vi "Set Controls from String Formats_ArrayInputs_SignalingValue.vi"(4 "Defer Panel Updates (T)":bool=TRUE, 6 "Disabled":u8[](array[numeric]), 7 "milliseconds to wait (10 ms)":u32=10, 8 "error in (no error)":errorcluster, 9 "Values":string[](array[string]), 10 "Labels":string[](array[string]), 11 "VI Server Cluster":T1) -> (0 "error out":errorcluster, 3 "VI Server Cluster.DUP":T1)   [LabVIEW 2020, in "VI Server Toolkit LV2013.lvlib"]
doc: "Set multiple Controls Value from string format and converts string values of the selected GUI objects onto original data type."
uses:
  VI Server Toolkit LV2013.lvlib
  VI Server_TypeDefs/VI Server_RefsCluster.ctl
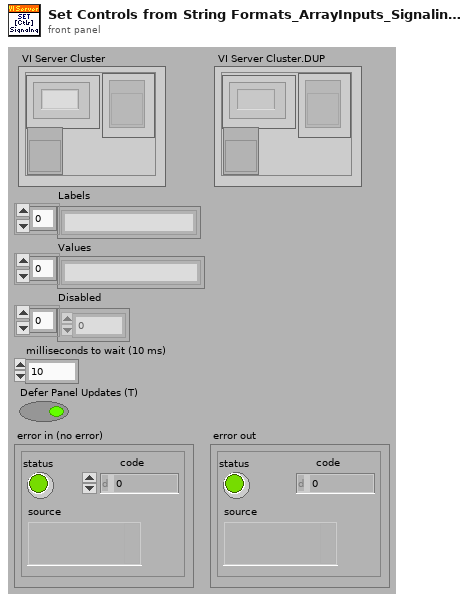
[diagram p1: front panel]
types:
  T1 = typedef "VI Server_RefsCluster.ctl" = cluster{"Labels":string[], "Refs":refnum<vi>[], "VI Ref":refnum<vi>}
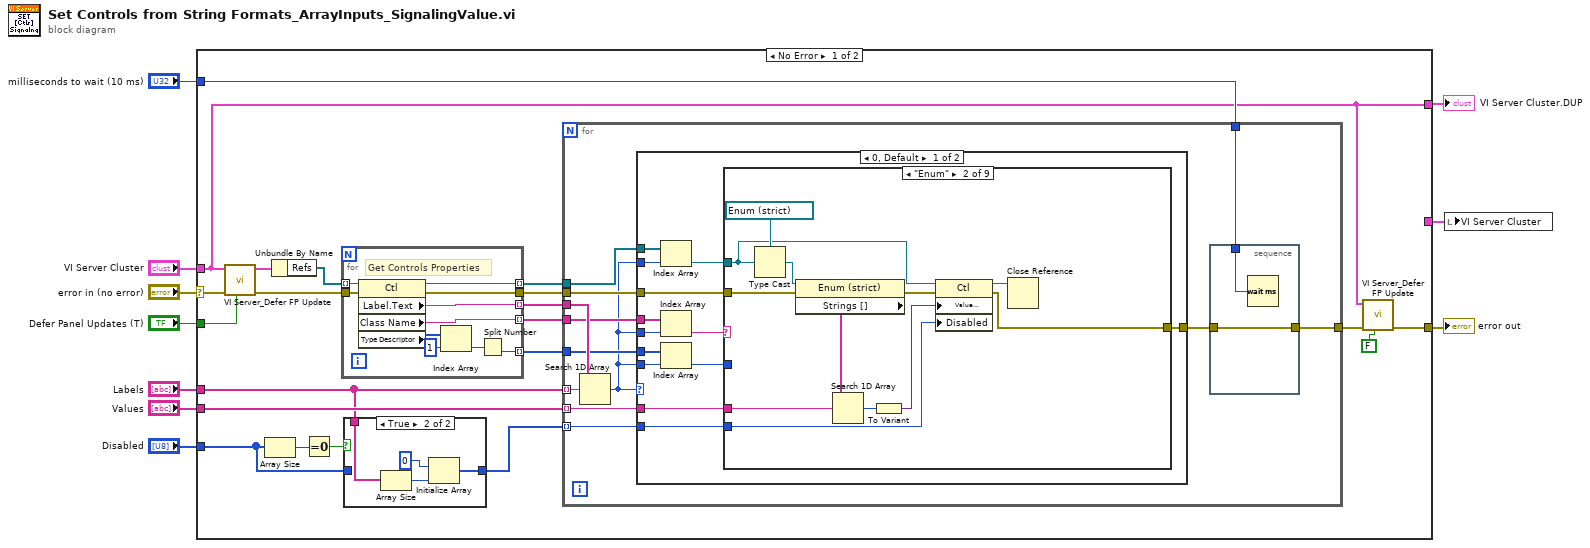
[diagram p0: block diagram]
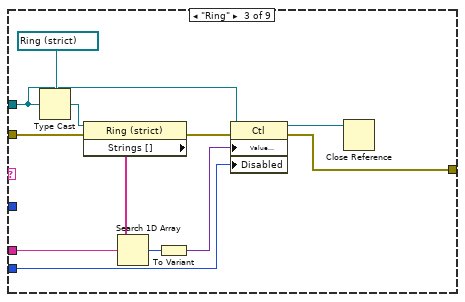
[diagram p4: hidden frame]
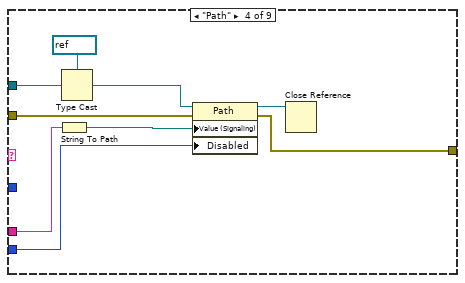
[diagram p5: hidden frame]
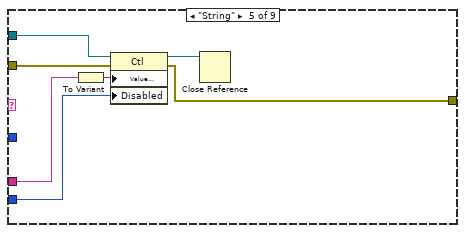
[diagram p6: hidden frame]
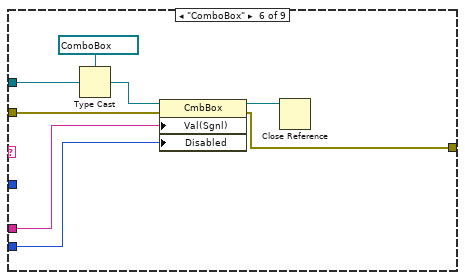
[diagram p7: hidden frame]
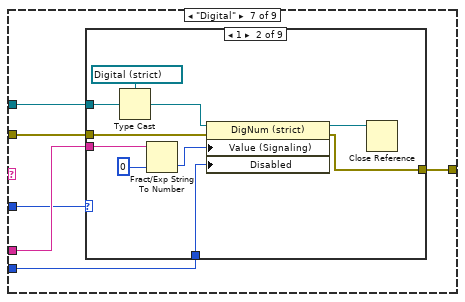
[diagram p8: hidden frame]
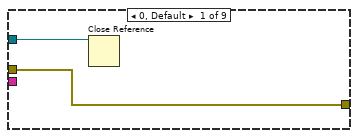
[diagram p9: hidden frame]
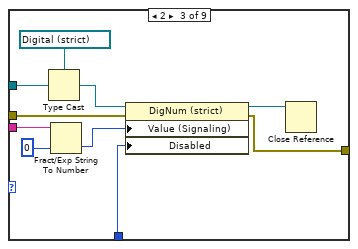
[diagram p10: hidden frame]
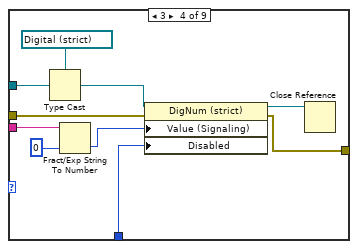
[diagram p11: hidden frame]
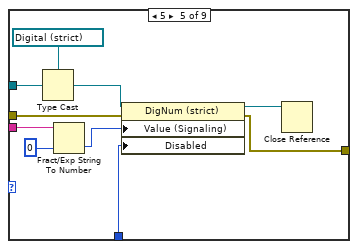
[diagram p12: hidden frame]
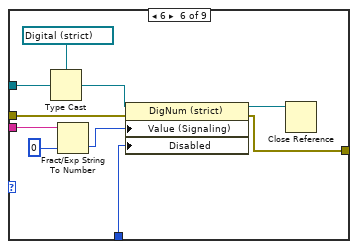
[diagram p13: hidden frame]
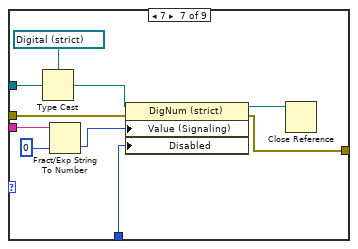
[diagram p14: hidden frame]
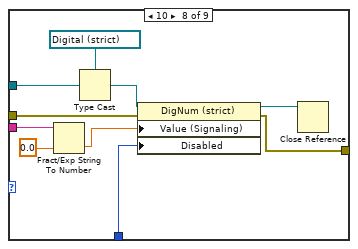
[diagram p15: hidden frame]
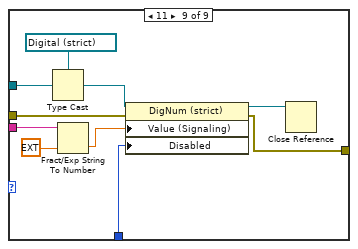
[diagram p16: hidden frame]
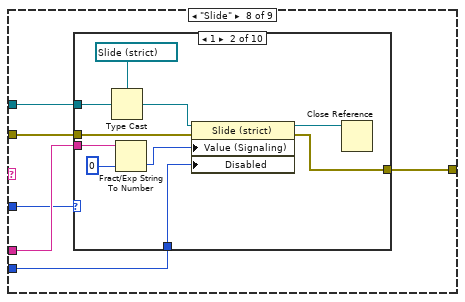
[diagram p17: hidden frame]
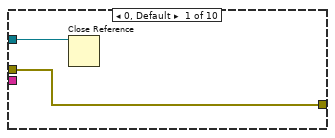
[diagram p18: hidden frame]
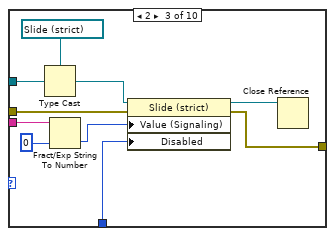
[diagram p19: hidden frame]
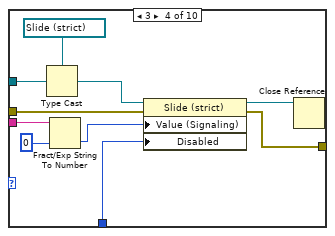
[diagram p20: hidden frame]
diagram:
  n1 = case shown="No Error" "error in (no error)" {
    selector: "error in (no error)" -> [w19 w324]
    tunnel: "Labels" -> [w21 _]
    tunnel: "Disabled" -> [w31 _]
    tunnel: "Values" -> [w22 _]
    tunnel: [w16 w324] -> w7
    tunnel: "VI Server Cluster" -> [w11 _]
    tunnel: [w11 _] -> w3
    tunnel: "milliseconds to wait (10 ms)" -> [w13 _]
    tunnel: "Defer Panel Updates (T)" -> [w12 _]
    tunnel: [_ w323] -> w1
    frame No Error {
      n2 = call "VI Server_Defer FP Update.vi"("Defer Panel Updates? (F)"=w12, "error in"=w19, "VI Server Cluster"=w11) -> ("error out"=w18:errorcluster, "VI Server Cluster.DUP"=w17:T1)  [unwired: 7 out]
      n3 = Array Size(array=w31) -> (size(s)=w25:i32)
      n4 = Unbundle By Name(w17) -> ("Refs"=w20:refnum<vi>[])
      n5 = Equal To 0?(x=w25) -> (x = 0?=w24:bool)
      n6 = for {
        tunnel: w20 -> [w322] mode=indexing
        tunnel: w18 -> [w321]
        tunnel: [w320] -> w30 mode=indexing
        tunnel: [w319] -> w28 mode=indexing
        tunnel: [w318] -> w29 mode=indexing
        tunnel: [w317] -> w27
        tunnel: [w313] -> w26 mode=indexing
        # "Get Controls Properties"
        n7 = property class="Ctl"(reference=w322, error in=w321) -> (reference out=w318:refnum<vi>, error out=w317:errorcluster, "Label.Text"=w320:string, "Class Name"=w319:string, "Type Descriptor"=w316:i16[])
        n8 = Index Array(array=w316, index=1) -> (element=w314:i16)
        n9 = Split Number(x=w314) -> (lo(x)=w313:u8)  [unwired: 1 out]
      }
      n10 = case shown="True" w24 {
        tunnel: w31 -> [w32 _]
        tunnel: [w32 w33] -> w23
        tunnel: w21 -> [_ w34]
        frame False {
        }
        frame True {
          n11 = Array Size(array=w34) -> (size(s)=w36:i32)
          n12 = Initialize Array(u8 0, w36) -> (w33:u8[])
        }
      }
      n13 = for {
        tunnel: w21 -> [w46] mode=indexing
        tunnel: w30 -> [w48]
        tunnel: w29 -> [w44]
        tunnel: w28 -> [w47]
        tunnel: w22 -> [w45] mode=indexing
        tunnel: w27 -> [w43]
        tunnel: [w38] -> w15
        tunnel: w26 -> [w42]
        tunnel: w23 -> [w40] mode=indexing
        tunnel: w13 -> [w37]
        n14 = Search 1D Array(1D array=w48, element=w46) -> (index of element=w41:i32)  [unwired: 1 out]
        n15 = case shown="0, Default" w41 {
          tunnel: w44 -> [w63 _]
          tunnel: w41 -> [w62 _]
          tunnel: w47 -> [w61 _]
          tunnel: w41 -> [w60 _]
          tunnel: w45 -> [w57 _]
          tunnel: w43 -> [w56 w312]
          tunnel: [w55 w312] -> w39
          tunnel: w42 -> [w54 _]
          tunnel: w41 -> [w53 _]
          tunnel: w40 -> [w51 _]
          frame 0, Default {
            n16 = Index Array(array=w63, index=w62) -> (element=w58:refnum<vi>)
            n17 = Index Array(array=w61, index=w60) -> (element=w59:string)
            n18 = Index Array(array=w54, index=w53) -> (element=w52:u8)
            n19 = case shown="\"Enum\"" w59 {
              tunnel: w58 -> [_ w68 w78 w92 w104 w112 w116 w204 w309]
              tunnel: w57 -> [_ w74 w87 w96 w103 w105 w115 w203 w299]
              tunnel: w56 -> [w64 w71 w81 w93 w101 w110 w118 w206 w311]
              tunnel: [w64 w69 w79 w94 w100 w109 w117 w205 w310] -> w55
              tunnel: w52 -> [_ _ _ _ _ _ w114 w202 _]
              tunnel: w51 -> [_ w65 w77 w89 w99 w108 w113 w201 w307]
              frame "", Default {
              }
              frame "Enum" {
                n20 = Type Cast(type=refnum<vi> refnum ("Enum"), x=w68) -> (*(type *) &x=w75:refnum<vi>)
                n21 = property class="Enum (strict)"(reference=w75, error in=w71) -> (error out=w70:errorcluster, "Strings []"=w73:string[])  [unwired: 1 out]
                n22 = Search 1D Array(1D array=w73, element=w74) -> (index of element=w67:i32)  [unwired: 1 out]
                n23 = To Variant(anything=w67) -> (Variant=w66:variant)
                n24 = property class="Ctl"(reference=w68, error in=w70, "Value (Signaling)"=w66, "Disabled"=w65) -> (reference out=w72:refnum<vi>, error out=w69:errorcluster)
                n25 = Close Reference(reference=w72) -> ()  [unwired: 1 in, 1 out]
              }
              frame "Ring" {
                n26 = Type Cast(type=refnum<vi> refnum ("Ring"), x=w78) -> (*(type *) &x=w88:refnum<vi>)
                n27 = property class="Ring (strict)"(reference=w88, error in=w81) -> (error out=w80:errorcluster, "Strings []"=w85:string[])  [unwired: 1 out]
                n28 = Search 1D Array(1D array=w85, element=w87) -> (index of element=w86:i32)  [unwired: 1 out]
                n29 = To Variant(anything=w86) -> (Variant=w84:variant)
                n30 = property class="Ctl"(reference=w78, error in=w80, "Value (Signaling)"=w84, "Disabled"=w77) -> (reference out=w83:refnum<vi>, error out=w79:errorcluster)
                n31 = Close Reference(reference=w83) -> ()  [unwired: 1 in, 1 out]
              }
              frame "Path" {
                n32 = String To Path(string=w96) -> (path=w97:path)
                n33 = Type Cast(type=refnum<vi> refnum ("Path"), x=w92) -> (*(type *) &x=w91:refnum<vi>)
                n34 = property class="Path"(reference=w91, error in=w93, "Value (Signaling)"=w97, "Disabled"=w89) -> (reference out=w95:refnum<vi>, error out=w94:errorcluster)
                n35 = Close Reference(reference=w95) -> ()  [unwired: 1 in, 1 out]
              }
              frame "String" {
                n36 = To Variant(anything=w103) -> (Variant=w98:variant)
                n37 = property class="Ctl"(reference=w104, error in=w101, "Value (Signaling)"=w98, "Disabled"=w99) -> (reference out=w102:refnum<vi>, error out=w100:errorcluster)
                n38 = Close Reference(reference=w102) -> ()  [unwired: 1 in, 1 out]
              }
              frame "ComboBox" {
                n39 = Type Cast(type=refnum<vi> refnum ("TDS.TriggerType"), x=w112) -> (*(type *) &x=w107:refnum<vi>)
                n40 = property class="CmbBox"(reference=w107, error in=w110, "Val(Sgnl)"=w105, "Disabled"=w108) -> (reference out=w111:refnum<vi>, error out=w109:errorcluster)
                n41 = Close Reference(reference=w111) -> ()  [unwired: 1 in, 1 out]
              }
              frame "Digital" {
                n42 = case shown="1" w114 {
                  tunnel: w118 -> [w120 w130 w137 w144 w156 w164 w177 w184 w197]
                  tunnel: [w120 w129 w134 w147 w158 w167 w174 w187 w196] -> w117
                  tunnel: w116 -> [w119 w128 w140 w150 w160 w170 w180 w190 w200]
                  tunnel: w115 -> [_ w126 w136 w146 w155 w165 w176 w185 w195]
                  tunnel: w113 -> [_ w124 w138 w145 w154 w166 w175 w186 w194]
                  frame 0, Default {
                    n43 = Close Reference(reference=w119) -> ()  [unwired: 1 in, 1 out]
                  }
                  frame 1 {
                    n44 = Type Cast(type=refnum<vi> refnum ("I8"), x=w128) -> (*(type *) &x=w127:refnum<vi>)
                    n45 = Fract/Exp String To Number(string=w126, default (0 dbl)=i8 0) -> (number=w122:i8)  [unwired: 3 out]
                    n46 = property class="DigNum (strict)"(reference=w127, error in=w130, "Value (Signaling)"=w122, "Disabled"=w124) -> (reference out=w123:refnum<vi>, error out=w129:errorcluster)
                    n47 = Close Reference(reference=w123) -> ()  [unwired: 1 in, 1 out]
                  }
                  frame 2 {
                    n48 = Type Cast(type=refnum<vi> refnum ("I16"), x=w140) -> (*(type *) &x=w135:refnum<vi>)
                    n49 = Fract/Exp String To Number(string=w136, default (0 dbl)=i16 0) -> (number=w132:i16)  [unwired: 3 out]
                    n50 = property class="DigNum (strict)"(reference=w135, error in=w137, "Value (Signaling)"=w132, "Disabled"=w138) -> (reference out=w133:refnum<vi>, error out=w134:errorcluster)
                    n51 = Close Reference(reference=w133) -> ()  [unwired: 1 in, 1 out]
                  }
                  frame 3 {
                    n52 = Type Cast(type=refnum<vi> refnum ("I32"), x=w150) -> (*(type *) &x=w148:refnum<vi>)
                    n53 = Fract/Exp String To Number(string=w146, default (0 dbl)=0) -> (number=w142:i32)  [unwired: 3 out]
                    n54 = property class="DigNum (strict)"(reference=w148, error in=w144, "Value (Signaling)"=w142, "Disabled"=w145) -> (reference out=w143:refnum<vi>, error out=w147:errorcluster)
                    n55 = Close Reference(reference=w143) -> ()  [unwired: 1 in, 1 out]
                  }
                  frame 5 {
                    n56 = Type Cast(type=refnum<vi> refnum ("U8"), x=w160) -> (*(type *) &x=w157:refnum<vi>)
                    n57 = Fract/Exp String To Number(string=w155, default (0 dbl)=u8 0) -> (number=w152:u8)  [unwired: 3 out]
                    n58 = property class="DigNum (strict)"(reference=w157, error in=w156, "Value (Signaling)"=w152, "Disabled"=w154) -> (reference out=w153:refnum<vi>, error out=w158:errorcluster)
                    n59 = Close Reference(reference=w153) -> ()  [unwired: 1 in, 1 out]
                  }
                  frame 6 {
                    n60 = Type Cast(type=refnum<vi> refnum ("U16"), x=w170) -> (*(type *) &x=w168:refnum<vi>)
                    n61 = Fract/Exp String To Number(string=w165, default (0 dbl)=u16 0) -> (number=w162:u16)  [unwired: 3 out]
                    n62 = property class="DigNum (strict)"(reference=w168, error in=w164, "Value (Signaling)"=w162, "Disabled"=w166) -> (reference out=w163:refnum<vi>, error out=w167:errorcluster)
                    n63 = Close Reference(reference=w163) -> ()  [unwired: 1 in, 1 out]
                  }
                  frame 7 {
                    n64 = Type Cast(type=refnum<vi> refnum ("U32"), x=w180) -> (*(type *) &x=w178:refnum<vi>)
                    n65 = Fract/Exp String To Number(string=w176, default (0 dbl)=u32 0) -> (number=w172:u32)  [unwired: 3 out]
                    n66 = property class="DigNum (strict)"(reference=w178, error in=w177, "Value (Signaling)"=w172, "Disabled"=w175) -> (reference out=w173:refnum<vi>, error out=w174:errorcluster)
                    n67 = Close Reference(reference=w173) -> ()  [unwired: 1 in, 1 out]
                  }
                  frame 10 {
                    n68 = Fract/Exp String To Number(string=w185, default (0 dbl)=0.0) -> (number=w182:dbl)  [unwired: 3 out]
                    n69 = Type Cast(type=refnum<vi> refnum ("DBL"), x=w190) -> (*(type *) &x=w188:refnum<vi>)
                    n70 = property class="DigNum (strict)"(reference=w188, error in=w184, "Value (Signaling)"=w182, "Disabled"=w186) -> (reference out=w183:refnum<vi>, error out=w187:errorcluster)
                    n71 = Close Reference(reference=w183) -> ()  [unwired: 1 in, 1 out]
                  }
                  frame 11 {
                    n72 = Type Cast(type=refnum<vi> refnum ("EXT"), x=w200) -> (*(type *) &x=w198:refnum<vi>)
                    n73 = Fract/Exp String To Number(string=w195, default (0 dbl)=ext 0.0) -> (number=w192:ext)  [unwired: 3 out]
                    n74 = property class="DigNum (strict)"(reference=w198, error in=w197, "Value (Signaling)"=w192, "Disabled"=w194) -> (reference out=w193:refnum<vi>, error out=w196:errorcluster)
                    n75 = Close Reference(reference=w193) -> ()  [unwired: 1 in, 1 out]
                  }
                }
              }
              frame "Slide" {
                n76 = case shown="1" w202 {
                  tunnel: w206 -> [w208 w215 w226 w234 w245 w254 w265 w275 w285 w295]
                  tunnel: [w208 w216 w227 w236 w243 w255 w262 w272 w282 w292] -> w205
                  tunnel: w204 -> [w207 w218 w228 w238 w248 w258 w268 w278 w288 w298]
                  tunnel: w203 -> [_ w214 w223 w233 w244 w253 w264 w274 w284 w294]
                  tunnel: w201 -> [_ w213 w224 w232 w242 w252 w263 w273 w283 w293]
                  frame 0, Default {
                    n77 = Close Reference(reference=w207) -> ()  [unwired: 1 in, 1 out]
                  }
                  frame 1 {
                    n78 = Type Cast(type=refnum<vi> refnum ("Slide"), x=w218) -> (*(type *) &x=w217:refnum<vi>)
                    n79 = Fract/Exp String To Number(string=w214, default (0 dbl)=u8 0) -> (number=w209:u8)  [unwired: 3 out]
                    n80 = property class="Slide (strict)"(reference=w217, error in=w215, "Value (Signaling)"=w209, "Disabled"=w213) -> (reference out=w211:refnum<vi>, error out=w216:errorcluster)
                    n81 = Close Reference(reference=w211) -> ()  [unwired: 1 in, 1 out]
                  }
                  frame 2 {
                    n82 = Type Cast(type=refnum<vi> refnum ("Slide"), x=w228) -> (*(type *) &x=w225:refnum<vi>)
                    n83 = Fract/Exp String To Number(string=w223, default (0 dbl)=u16 0) -> (number=w220:u16)  [unwired: 3 out]
                    n84 = property class="Slide (strict)"(reference=w225, error in=w226, "Value (Signaling)"=w220, "Disabled"=w224) -> (reference out=w221:refnum<vi>, error out=w227:errorcluster)
                    n85 = Close Reference(reference=w221) -> ()  [unwired: 1 in, 1 out]
                  }
                  frame 3 {
                    n86 = Type Cast(type=refnum<vi> refnum ("Slide"), x=w238) -> (*(type *) &x=w235:refnum<vi>)
                    n87 = Fract/Exp String To Number(string=w233, default (0 dbl)=0) -> (number=w230:i32)  [unwired: 3 out]
                    n88 = property class="Slide (strict)"(reference=w235, error in=w234, "Value (Signaling)"=w230, "Disabled"=w232) -> (reference out=w231:refnum<vi>, error out=w236:errorcluster)
                    n89 = Close Reference(reference=w231) -> ()  [unwired: 1 in, 1 out]
                  }
                  frame 5 {
                    n90 = Fract/Exp String To Number(string=w244, default (0 dbl)=u8 0) -> (number=w240:u8)  [unwired: 3 out]
                    n91 = Type Cast(type=refnum<vi> refnum ("Slide"), x=w248) -> (*(type *) &x=w246:refnum<vi>)
                    n92 = property class="Slide (strict)"(reference=w246, error in=w245, "Value (Signaling)"=w240, "Disabled"=w242) -> (reference out=w241:refnum<vi>, error out=w243:errorcluster)
                    n93 = Close Reference(reference=w241) -> ()  [unwired: 1 in, 1 out]
                  }
                  frame 6 {
                    n94 = Type Cast(type=refnum<vi> refnum ("Slide"), x=w258) -> (*(type *) &x=w256:refnum<vi>)
                    n95 = Fract/Exp String To Number(string=w253, default (0 dbl)=u16 0) -> (number=w250:u16)  [unwired: 3 out]
                    n96 = property class="Slide (strict)"(reference=w256, error in=w254, "Value (Signaling)"=w250, "Disabled"=w252) -> (reference out=w251:refnum<vi>, error out=w255:errorcluster)
                    n97 = Close Reference(reference=w251) -> ()  [unwired: 1 in, 1 out]
                  }
                  frame 7 {
                    n98 = Type Cast(type=refnum<vi> refnum ("Slide"), x=w268) -> (*(type *) &x=w266:refnum<vi>)
                    n99 = Fract/Exp String To Number(string=w264, default (0 dbl)=u32 0) -> (number=w260:u32)  [unwired: 3 out]
                    n100 = property class="Slide (strict)"(reference=w266, error in=w265, "Value (Signaling)"=w260, "Disabled"=w263) -> (reference out=w261:refnum<vi>, error out=w262:errorcluster)
                    n101 = Close Reference(reference=w261) -> ()  [unwired: 1 in, 1 out]
                  }
                  frame 9 {
                    n102 = Type Cast(type=refnum<vi> refnum ("Slide"), x=w278) -> (*(type *) &x=w276:refnum<vi>)
                    n103 = Fract/Exp String To Number(string=w274, default (0 dbl)=sgl 0.0) -> (number=w270:sgl)  [unwired: 3 out]
                    n104 = property class="Slide (strict)"(reference=w276, error in=w275, "Value (Signaling)"=w270, "Disabled"=w273) -> (reference out=w271:refnum<vi>, error out=w272:errorcluster)
                    n105 = Close Reference(reference=w271) -> ()  [unwired: 1 in, 1 out]
                  }
                  frame 10 {
                    n106 = Fract/Exp String To Number(string=w284, default (0 dbl)=0.0) -> (number=w280:dbl)  [unwired: 3 out]
                    n107 = Type Cast(type=refnum<vi> refnum ("Slide"), x=w288) -> (*(type *) &x=w286:refnum<vi>)
                    n108 = property class="Slide (strict)"(reference=w286, error in=w285, "Value (Signaling)"=w280, "Disabled"=w283) -> (reference out=w281:refnum<vi>, error out=w282:errorcluster)
                    n109 = Close Reference(reference=w281) -> ()  [unwired: 1 in, 1 out]
                  }
                  frame 11 {
                    n110 = Fract/Exp String To Number(string=w294, default (0 dbl)=ext 0.0) -> (number=w290:ext)  [unwired: 3 out]
                    n111 = Type Cast(type=refnum<vi> refnum ("Slide"), x=w298) -> (*(type *) &x=w296:refnum<vi>)
                    n112 = property class="Slide (strict)"(reference=w296, error in=w295, "Value (Signaling)"=w290, "Disabled"=w293) -> (reference out=w291:refnum<vi>, error out=w292:errorcluster)
                    n113 = Close Reference(reference=w291) -> ()  [unwired: 1 in, 1 out]
                  }
                }
              }
              frame "Boolean" {
                n114 = Type Cast(type=refnum<vi> refnum ("Boolean 2"), x=w309) -> (*(type *) &x=w308:refnum<vi>)
                n115 = Equal?(x=w299, y="TRUE" ("x")) -> (x = y?=w301:bool)
                n116 = Equal?(x=w299, y="ON" ("x")) -> (x = y?=w302:bool)
                n117 = Or(x=w301, y=w302) -> (x .or. y?=w300:bool)
                n118 = property class="Bool (strict)"(reference=w308, error in=w311, "Value (Signaling)"=w300, "Disabled"=w307) -> (reference out=w305:refnum<vi>, error out=w310:errorcluster)
                n119 = Close Reference(reference=w305) -> ()  [unwired: 1 in, 1 out]
              }
            }
          }
          frame -1 {
          }
        }
        n120 = stacked-sequence {
          tunnel: w39 -> [w50]
          tunnel: [w50] -> w38
          tunnel: w37 -> [w49]
          frame #0 {
            n121 = Wait (ms)(milliseconds to wait=w49) -> ()  [unwired: 1 out]
          }
        }
      }
      n122 = call "VI Server_Defer FP Update.vi"("Defer Panel Updates? (F)"=FALSE ("Defer Panel Updates (F)"), "error in"=w15, "VI Server Cluster"=w11) -> ("error out"=w16:errorcluster)  [unwired: 8 out]
    }
    frame Error {
      n123 = call "VI Server_Empty VI Server Cluster.vi"() -> ("VI Server Cluster"=w323:T1)  [unwired: 7 in]
    }
  }
  "error out" <- w7
  "VI Server Cluster.DUP" <- w3
  n124 = local write "VI Server Cluster"(w1) -> ()
